vi "2 D Array Sum.vi"() -> ()   [LabVIEW 2015]
panel:
  out "Total sum":i32
  out "Sum of 2 D array":i32[](array[numeric])
  out "Tables":i32[][](array[numeric])
  # "2 D Array Sum"
  # "Pardeep Kumar"
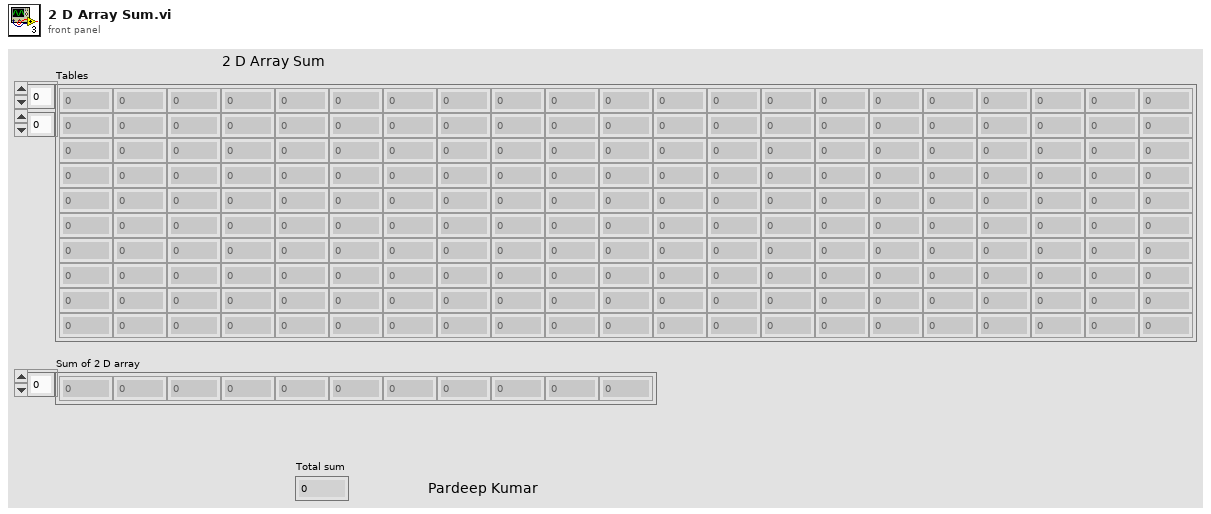
[diagram p1: front panel]
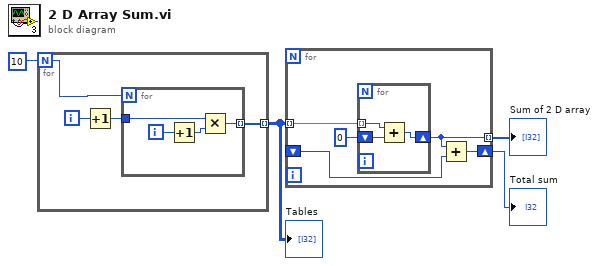
[diagram p0: block diagram]
diagram:
  n1 = for {
    N: 10 -> [w6]
    tunnel: [w5] -> w3 mode=indexing
    i -> [w8]
    n2 = Increment(x=w8) -> (x+1=w7:i32)
    n3 = for {
      N: w6 -> [_]
      tunnel: w7 -> [w12]
      tunnel: [w9] -> w5 mode=indexing
      i -> [w10]
      n4 = Increment(x=w10) -> (x+1=w11:i32)
      n5 = Multiply(x=w12, y=w11) -> (x*y=w9:i32)
    }
  }
  "Tables" <- w3
  n6 = for {
    tunnel: w3 -> [w17] mode=indexing
    tunnel: [w15] -> w2 mode=indexing
    shift-right: [w14] -> w1
    shift-left: _ -> [w13]
    n7 = for {
      tunnel: w17 -> [w20] mode=indexing
      shift-right: [w19] -> w15
      shift-left: 0 -> [w18]
      n8 = Add(x=w20, y=w18) -> (x+y=w19:i32)
    }
    n9 = Add(x=w15, y=w13) -> (x+y=w14:i32)
  }
  "Sum of 2 D array" <- w2
  "Total sum" <- w1
